vi "Local to Global Valve Numbers.vi"(0 "Reactor ID #":i32, 3 "List of Local Valves":i32[](array[numeric]), 4 "Valves Per Reactor":i32) -> (5 "List of Global Valves":i32[](array[numeric]))   [LabVIEW 2022 SP3]
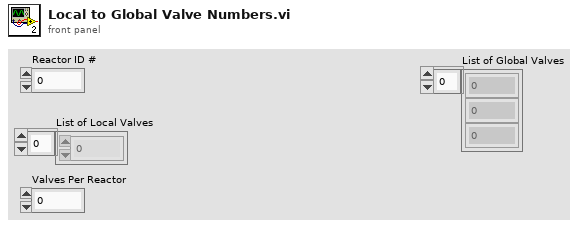
[diagram p1: front panel]
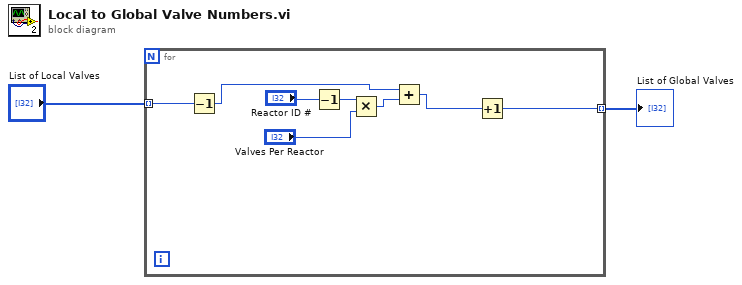
[diagram p0: block diagram]
diagram:
  n1 = for {
    tunnel: "List of Local Valves" -> [w10] mode=indexing
    tunnel: [w3] -> w1 mode=indexing
    n2 = Decrement(x=w10) -> (x-1=w5:i32)
    n3 = Decrement(x="Reactor ID #") -> (x-1=w8:i32)
    n4 = Multiply(x=w8, y="Valves Per Reactor") -> (x*y=w6:i32)
    n5 = Add(x=w5, y=w6) -> (x+y=w4:i32)
    n6 = Increment(x=w4) -> (x+1=w3:i32)
  }
  "List of Global Valves" <- w1
